vi "Create Directory.vi"(5 "Username":string, 6 "Password":string, 7 "Address":string, 8 "Error In":errorcluster) -> (0 "Error Out":errorcluster)   [LabVIEW 2018, in "Tests.lvlib" / "SFTP.lvlib"]
uses:
  SFTP.lvlib
  <vilib>/addons/_JKI Toolkits/Caraya/classes/Test/Test.lvclass
  <vilib>/addons/_JKI Toolkits/Caraya/classes/Assert/Assert.lvclass
  src/Toolkit/API/SFTP/SFTP.lvclass
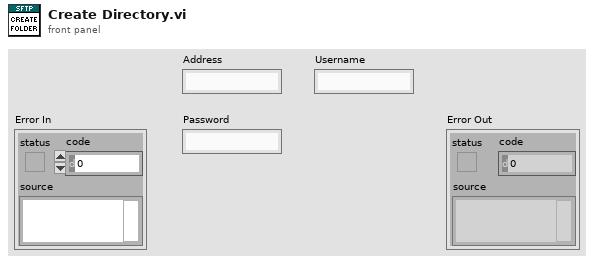
[diagram p1: front panel]
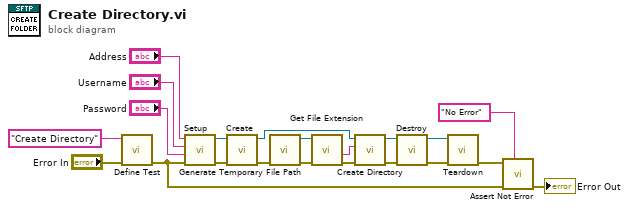
[diagram p0: block diagram]
diagram:
  n1 = call <vilib>:"Define Test.vi"("error in (no error)"="Error In", "Label (VI Title)"="Create Directory") -> ("error out"=w16:errorcluster)  [unwired: 9 in]
  n2 = call "Setup.vi"("Error In"=w16, "Password"="Password", "Username"="Username", "Address"="Address") -> ("Error Out"=w17:errorcluster, "Sesssion"=w12:refnum<class "Session.lvclass">)  [unwired: 6 in]
  n3 = call "Create.vi"("Error In"=w17, "Session"=w12) -> ("Error Out"=w8:errorcluster, "SFTP"=w3:refnum<class "SFTP.lvclass">)  [unwired: 8 in]
  n4 = call <vilib>:"Generate Temporary File Path.vi"("error in (no error)"=w8) -> ("error out"=w6:errorcluster, "Unique Temporary File Path"=w7:path)  [unwired: 9 in]
  n5 = call <vilib>:"Get File Extension.vi"("error in (no error)"=w6, "file"=w7) -> ("error out"=w5:errorcluster, "filename without extension"=w4:string)  [unwired: 5 in, 3 out]
  n6 = call "Create Directory.vi"("Error In"=w5, "Remote Path"=w4, "SFTP In"=w3) -> ("Error Out"=w2:errorcluster, "SFTP Out"=w1:refnum<class "SFTP.lvclass">)  [unwired: 7 in]
  n7 = call "Destroy.vi"("Error In"=w2, "SFTP"=w1) -> ("Error Out"=w11:errorcluster, "Session"=w9:refnum<class "Session.lvclass">)  [unwired: 8 in]
  n8 = call "Teardown.vi"("Error In"=w11, "Session"=w9) -> ("Error Out"=w10:errorcluster)  [unwired: 9 in]
  n9 = call <vilib>:"Assert Not Error.vi"("Label"="No Error", "error in (no error)"=w16, "Not Error?"=w10) -> ("error out"=→"Error Out":errorcluster)  [unwired: 8 in]
